vi "ExportResults.vi"(8 "error in (no error)":errorcluster, 11 "CDependencyInspector in":refnum<class "CDependencyInspection.lvclass">) -> (0 "error out":errorcluster, 3 "CDependencyInspector out":refnum<class "CDependencyInspection.lvclass">)   [LabVIEW 2020, in "DependencyInspection.lvlib" / "CDependencyInspection.lvclass"]
uses:
  CDependencyInspection.lvclass
  obj/Addons/LabVIEWObjectInterfaces.lvlibp/ErrorManager/ErrorManager/ErrorType.ctl
  obj/Addons/LabVIEWObjectInterfaces.lvlibp/LabVIEWObjectInterfaces/IErrorManager/IErrorManager.lvclass
  obj/Addons/ExtensionInterfaces.lvlibp/IExporter/ExportType.ctl
  obj/Addons/ExtensionInterfaces.lvlibp/IExporter/IExporter.lvclass
  obj/Addons/ErrorManager.lvlibp/ErrorManager/ErrorManager.lvclass
  CDependencyList/CDependencyList.lvclass
  CRuleList/CRuleList.lvclass
  CReporter/CReporter.lvclass
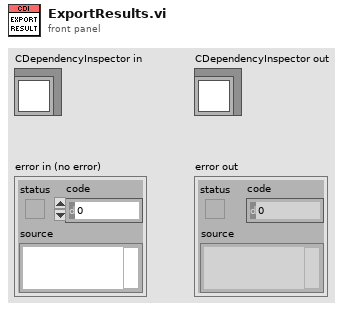
[diagram p1: front panel]
types:
  T1 = typedef "ExtensionInterfaces.lvlibp/IExporter.lvclass/ExportType.ctl" = enum16{"Dependencies", "Rules", "Invalid dependencies", "Concessions", "Undeclared"}
  T2 = typedef "LabVIEWObjectInterfaces.lvlibp/IErrorManager.lvclass/ErrorType.ctl" = enum16{"Info", "Warning", "Error"}
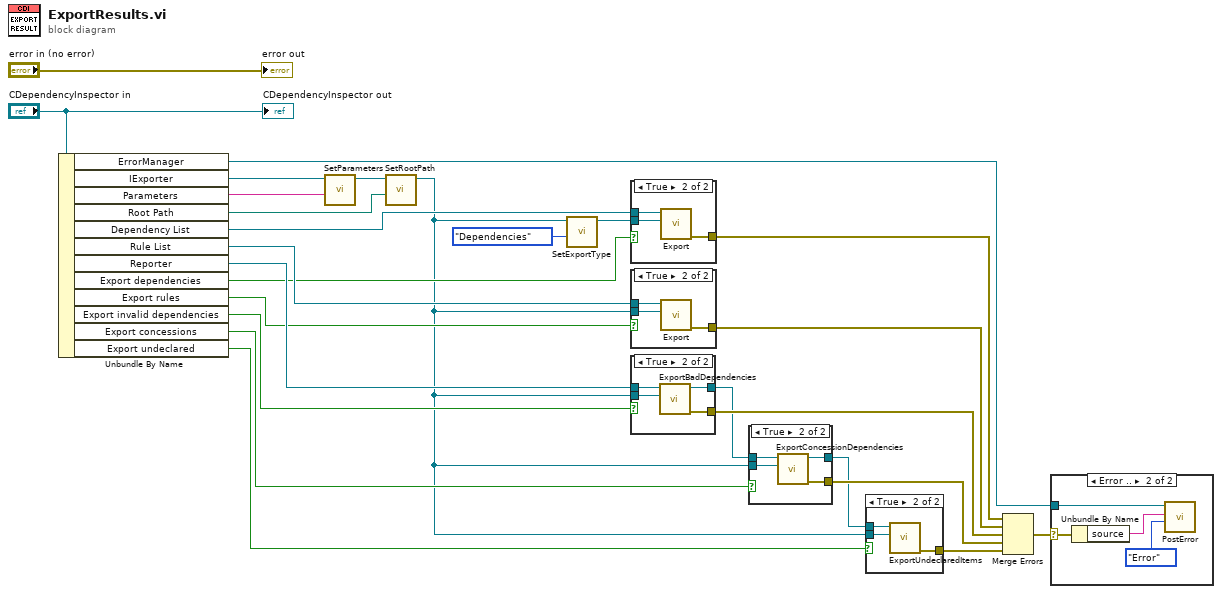
[diagram p0: block diagram]
diagram:
  n1 = Unbundle By Name("CDependencyInspector in") -> ("ErrorManager"=w20:refnum<class "ErrorManager.lvclass">, "IExporter"=w8:refnum<class "IExporter.lvclass">, "Parameters"=w7:string, "Root Path"=w5:path, "Dependency List"=w6:refnum<class "CDependencyList.lvclass">, "Rule List"=w25:refnum<class "CRuleList.lvclass">, "Reporter"=w16:refnum<class "CReporter.lvclass">, "Export dependencies"=w13:bool, "Export rules"=w12:bool, "Export invalid dependencies"=w11:bool, "Export concessions"=w10:bool, "Export undeclared"=w9:bool)
  n2 = call-dynamic "SetParameters.vi"("Parameters"=w7, "IExporter in"=w8) -> ("IExporter out"=w4:refnum<class "IExporter.lvclass">)  [unwired: 8 in, 1 out]
  n3 = call-dynamic "SetRootPath.vi"("Root path"=w5, "IExporter in"=w4) -> ("IExporter out"=w3:refnum<class "IExporter.lvclass">)  [unwired: 8 in, 1 out]
  n4 = call-dynamic "SetExportType.vi"("Export type"=ExportType."Dependencies", "IExporter in"=w3) -> ("IExporter out"=w2:refnum<class "IExporter.lvclass">)  [unwired: 8 in, 1 out]
  n5 = case shown="True" w13 {
    tunnel: w6 -> [_ w29]
    tunnel: [_ w28] -> w22
    tunnel: w2 -> [_ w27]
    frame False {
    }
    frame True {
      n6 = call-dynamic "Export.vi"("IExporter"=w27, "CDependencyList in"=w29) -> ("error out"=w28:errorcluster)  [unwired: 8 in, 1 out]
    }
  }
  n7 = case shown="True" w12 {
    tunnel: w25 -> [_ w32]
    tunnel: [_ w31] -> w23
    tunnel: w3 -> [_ w30]
    frame False {
    }
    frame True {
      n8 = call-dynamic "Export.vi"("IExporter"=w30, "CRuleList in"=w32) -> ("error out"=w31:errorcluster)  [unwired: 8 in, 1 out]
    }
  }
  n9 = case shown="True" w11 {
    tunnel: [_ w37] -> w19
    tunnel: w16 -> [w33 w36]
    tunnel: [w33 w35] -> w15
    tunnel: w3 -> [_ w34]
    frame False {
    }
    frame True {
      n10 = call-dynamic "ExportBadDependencies.vi"("IExporter"=w34, "CReporter in"=w36) -> ("error out"=w37:errorcluster, "CReporter out"=w35:refnum<class "CReporter.lvclass">)  [unwired: 8 in]
    }
  }
  n11 = case shown="True" w10 {
    tunnel: [_ w42] -> w17
    tunnel: w15 -> [w38 w41]
    tunnel: [w38 w40] -> w14
    tunnel: w3 -> [_ w39]
    frame False {
    }
    frame True {
      n12 = call-dynamic "ExportConcessionDependencies.vi"("IExporter"=w39, "CReporter in"=w41) -> ("error out"=w42:errorcluster, "CReporter out"=w40:refnum<class "CReporter.lvclass">)  [unwired: 8 in]
    }
  }
  n13 = case shown="True" w9 {
    tunnel: [_ w45] -> w18
    tunnel: w14 -> [_ w44]
    tunnel: w3 -> [_ w43]
    frame False {
    }
    frame True {
      n14 = call-dynamic "ExportUndeclaredItems.vi"("IExporter"=w43, "CReporter in"=w44) -> ("error out"=w45:errorcluster)  [unwired: 8 in, 1 out]
    }
  }
  n15 = Merge Errors(w22, w23, w19, w17, w18) -> (w21:errorcluster)
  n16 = case shown="Error .." w21 {
    selector: w21 -> [_ w48]
    tunnel: w20 -> [_ w49]
    frame No Error {
    }
    frame Error {
      n17 = Unbundle By Name(w48) -> ("source"=w47:string)
      n18 = call-dynamic "PostError.vi"("Type"=ErrorType."Error", "Message"=w47, "ErrorManager in"=w49) -> ()  [unwired: 7 in, 2 out]
    }
  }
  "error out" <- "error in (no error)"
  "CDependencyInspector out" <- "CDependencyInspector in"
